vi "PXI-Enumerate AO Channels.vi"() -> (1 "24-bit channels":tag[](array[tag]), 3 "AO.PhysicalChans":tag[](array[tag]))   [LabVIEW 2020]
uses:
  <resource>/objmgr/daqmx.rc
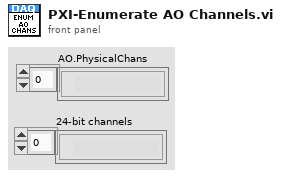
[diagram p1: front panel]
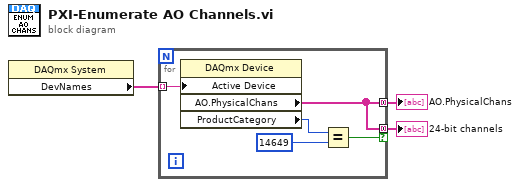
[diagram p0: block diagram]
diagram:
  n1 = property class="DAQmx System"() -> ("DevNames"=w2:tag[])  [unwired: 2 in, 2 out]
  n2 = for {
    tunnel: w2 -> [w8] mode=indexing
    tunnel: [w5] -> w3 mode=concatenating
    tunnel: [w5] -> w1 mode=concatenating if=w4
    n3 = property class="DAQmx Device"("Active Device"=w8) -> ("AO.PhysicalChans"=w5:tag[], "ProductCategory"=w6:i32)  [unwired: 2 in, 2 out]
    n4 = Equal?(x=w6, y=14649) -> (x = y?=w4:bool)
  }
  "AO.PhysicalChans" <- w3
  "24-bit channels" <- w1
